vi "市电监测-自动重合闸.vi"() -> ()   [LabVIEW 2016, in "环境动力监测库.lvlib" / "自动重合闸库.lvlib"]
uses:
  <vilib>/Utility/miscctls.llb/LVPointTypeDef.ctl
panel:
  out "data":T1
  out "x+1":u32
  in  "解除告警":bool
  out "日用电量":dbl format="%#.1f"
  out "小时用电量":dbl format="%#.1f"
  in  "清零":bool
  out "累计用电量":dbl format="%#.1f"
  out "漏电报警累加值":u16 caption="漏电报警次数"
  out "当前报警状态":u16(ring) items=["无报警"=0, "过压报警"=1, "欠压报警"=2, "过流报警"=4, "漏电报警"=8]
  out "通讯状态":u16(ring) items=["正常", "异常"]
  out "过流报警累加值":u16 caption="过流报警次数"
  out "欠压报警累加值":u16 caption="欠压报警次数"
  out "过压报警累加值":u16 caption="过压报警次数"
  out "当前漏电电流":dbl
  out "当前电流":dbl
  out "当前电压":u16
  # "市电监测/自动重合闸"
  # "V"
  # "A"
  # "mA"
  # "KW·h"
  # "KW·h"
  # "KW·h"
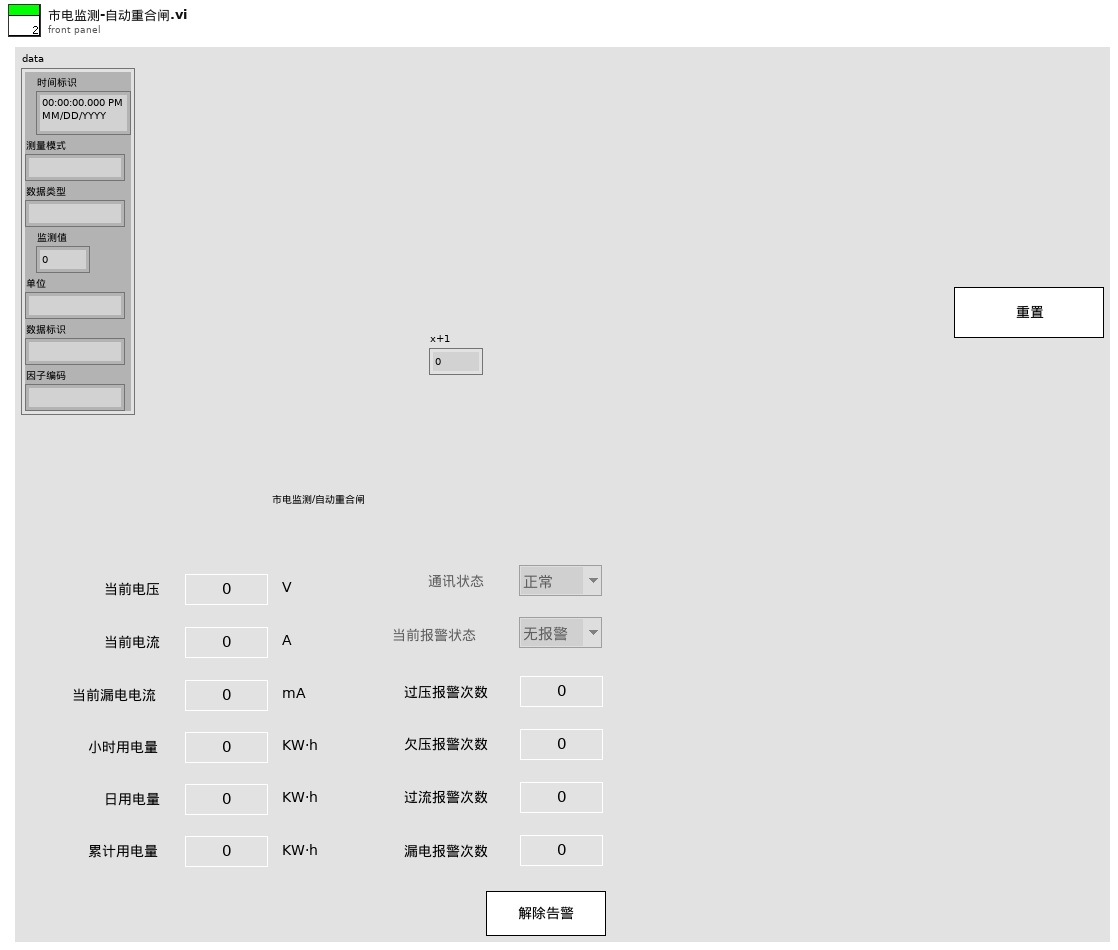
[diagram p1: front panel]
types:
  T1 = cluster{"时间标识":timestamp, "测量模式":string, "数据类型":string, "监测值":sgl, "单位":string, "数据标识":string, "因子编码":string}
  T2 = typedef "LVPointTypeDef.ctl" = cluster{"Horizontal":i16, "Vertical":i16}
  T3 = cluster{"监测项描述:输出":string, "端口":enum16{"AI0", "AI1", "AI2", "AI3", "AI4", "DI0", "DI1", "DI2", "DI3", "DI4", "DI5", "DI6", "DI7", "DO0", "DO1", "DO2", "DO3", "DO4", "DO5", "DO6", "DO7", "X0", "X1", "X2", "X3", "X4", "X5", "X6", "X7", "X8", "X9", "X10", "X11", "X12", "X13", "X14", "X15", "X16", "X17", "X18", "X19", "X20", "X21", "X22", "X23", "Y0", "Y1", "Y2", "Y3", "Y4", "Y5", "Y6", "Y7", "Y8", "Y9", "Y10", "Y11", "Y12", "Y13", "Y14", "Y15", "Y16", "Y17", "Y18", "Y19", "Y20", "Y21", "Y22", "Y23", "Y24", "Y25", "Y26", "Y27", "Y28", "Y29", "Y30", "Y31", "Y32", "Y33", "Y34", "Y35", "Y36", "Y37", "Y38", "Y39"}, "告警方式":enum32{"禁用告警", "闭合告警", "断开告警"}, "传感器型号":enum16{"PLC", "ZLAN", "ART"}, "声光告警启用":bool}
  T4 = enum16{"AI0", "AI1", "AI2", "AI3", "AI4", "DI0", "DI1", "DI2", "DI3", "DI4", "DI5", "DI6", "DI7", "DO0", "DO1", "DO2", "DO3", "DO4", "DO5", "DO6", "DO7", "X0", "X1", "X2", "X3", "X4", "X5", "X6", "X7", "X8", "X9", "X10", "X11", "X12", "X13", "X14", "X15", "X16", "X17", "X18", "X19", "X20", "X21", "X22", "X23", "Y0", "Y1", "Y2", "Y3", "Y4", "Y5", "Y6", "Y7", "Y8", "Y9", "Y10", "Y11", "Y12", "Y13", "Y14", "Y15", "Y16", "Y17", "Y18", "Y19", "Y20", "Y21", "Y22", "Y23", "Y24", "Y25", "Y26", "Y27", "Y28", "Y29", "Y30", "Y31", "Y32", "Y33", "Y34", "Y35", "Y36", "Y37", "Y38", "Y39"}
  T5 = cluster{"状态":cluster{"R0":i16, "R1":i16, "R2":i16, "R3":i16, "R4":i16, "R5":i16, "R6":i16, "R7":i16, "R8":i16, "R9":i16, "R10":i16, "R11":i16, "R12":i16, "R13":i16, "R14":i16, "R15":i16, "R16":i16, "R17":i16, "R18":i16, "R19":i16, "R20":i16, "R21":i16, "R22":i16, "R23":i16, "R24":i16, "R25":i16, "R26":i16, "R27":i16, "R28":i16, "R29":i16, "R30":i16, "R31":i16, "R32":i16, "R33":i16, "R34":i16, "R35":i16, "R36":i16, "R37":i16, "R38":i16, "R39":i16}, "输入状态":bool[], "输出状态":bool[], "参数设置":cluster{"R100":i16, "R101":i16, "R102":i16, "R103":i16, "R104":i16, "R105":i16, "R106":i16, "R107":i16, "R108":i16, "R109":i16, "R110":i16, "R111":i16, "R112":i16, "R113":i16, "R114":i16, "R115":i16, "R116":i16, "R117":i16, "R118":i16, "R119":i16, "R120":i16, "R121":i16, "R122":i16, "R123":i16}, "转换值":cluster{"AD0":sgl, "AD1":sgl, "AD2":sgl, "AD3":sgl, "AD4":sgl, "AD5":sgl}}
  T6 = cluster{"R0":i16, "R1":i16, "R2":i16, "R3":i16, "R4":i16, "R5":i16, "R6":i16, "R7":i16, "R8":i16, "R9":i16, "R10":i16, "R11":i16, "R12":i16, "R13":i16, "R14":i16, "R15":i16, "R16":i16, "R17":i16, "R18":i16, "R19":i16, "R20":i16, "R21":i16, "R22":i16, "R23":i16, "R24":i16, "R25":i16, "R26":i16, "R27":i16, "R28":i16, "R29":i16, "R30":i16, "R31":i16, "R32":i16, "R33":i16, "R34":i16, "R35":i16, "R36":i16, "R37":i16, "R38":i16, "R39":i16}
  T7 = typedef "采配水类型.ctl" = enum16{"V1", "V2", "V3", "V4", "室内V1", "室内V2", "固定站V1", "固定站V2", "浮船V1", "浮船V2", "养殖尾水", "广东华南所"}
  T8 = cluster{"状态":cluster{"R0":i16, "R1":i16, "R2":i16, "R3":i16, "R4":i16, "R5":i16, "R6":i16, "R7":i16, "R8":i16, "R9":i16, "R10":i16, "R11":i16, "R12":i16, "R13":i16, "R14":i16, "R15":i16, "R16":i16, "R17":i16, "R18":i16, "R19":i16, "R20":i16, "R21":i16, "R22":i16, "R23":i16, "R24":i16, "R25":i16, "R26":i16, "R27":i16, "R28":i16, "R29":i16, "R30":i16, "R31":i16, "R32":i16, "R33":i16, "R34":i16, "R35":i16, "R36":i16, "R37":i16, "R38":i16, "R39":i16, "R40":i16, "R41":i16, "R42":i16, "R43":i16, "R44":i16, "R45":i16, "R46":i16, "R47":i16, "R48":i16, "R49":i16, "R50":i16, "R51":i16, "R52":i16, "R53":i16, "R54":i16, "R55":i16, "R56":i16, "R57":i16, "R58":i16, "R59":i16, "R60":i16, "R61":i16, "R62":i16, "R63":i16, "R64":i16, "R65":i16, "R66":i16, "R67":i16, "R68":i16, "R69":i16}, "输入状态":bool[], "输出状态":bool[], "报警簇":bool[], "参数设置":cluster{"R100":i16, "R101":i16, "R102":i16, "R103":i16, "R104":i16, "R105":i16, "R106":i16, "R107":i16, "R108":i16, "R109":i16, "R110":i16, "R111":i16, "R112":i16, "R113":i16, "R114":i16, "R115":i16, "R116":i16, "R117":i16, "R118":i16, "R119":i16, "R120":i16, "R121":i16, "R122":i16, "R123":i16, "R124":i16}, "转换值":cluster{"AD0":sgl, "AD1":sgl, "AD2":sgl, "AD3":sgl, "AD4":sgl, "AD5":sgl}, "看门狗启用":bool, "氨氮模块名称":string, "总磷模块名称":string, "采配水模块类型":T7}
  T9 = cluster{"R0":i16, "R1":i16, "R2":i16, "R3":i16, "R4":i16, "R5":i16, "R6":i16, "R7":i16, "R8":i16, "R9":i16, "R10":i16, "R11":i16, "R12":i16, "R13":i16, "R14":i16, "R15":i16, "R16":i16, "R17":i16, "R18":i16, "R19":i16, "R20":i16, "R21":i16, "R22":i16, "R23":i16, "R24":i16, "R25":i16, "R26":i16, "R27":i16, "R28":i16, "R29":i16, "R30":i16, "R31":i16, "R32":i16, "R33":i16, "R34":i16, "R35":i16, "R36":i16, "R37":i16, "R38":i16, "R39":i16, "R40":i16, "R41":i16, "R42":i16, "R43":i16, "R44":i16, "R45":i16, "R46":i16, "R47":i16, "R48":i16, "R49":i16, "R50":i16, "R51":i16, "R52":i16, "R53":i16, "R54":i16, "R55":i16, "R56":i16, "R57":i16, "R58":i16, "R59":i16, "R60":i16, "R61":i16, "R62":i16, "R63":i16, "R64":i16, "R65":i16, "R66":i16, "R67":i16, "R68":i16, "R69":i16}
  T10 = cluster{"市电":cluster{"状态":bool, "电压:":u16, "电流：":dbl, "详情  ":bool}, "UPS":cluster{"状态":bool, "输入电压:":sgl, "输出电压:":sgl, "电池电量:":u8, "电量":u16, "详情  ":bool}, "蓄电池12V":cluster{"状态":bool, "电压:":sgl, "电流:":sgl, "电池电量:":u8, "电量":u16, "详情  ":bool, "充电":bool, "负载":bool}, "蓄电池24V":cluster{"状态":bool, "电压:":sgl, "电流:":sgl, "电池电量:":u8, "电量":u16, "详情  ":bool, "充电":bool, "负载":bool}}
  T11 = cluster{"漏水监测输出":cluster{"漏水监测告警":bool, "告警内容":string}, "门禁监测输出":cluster{"门禁监测告警":bool, "告警内容":string}, "门禁监测输出2":cluster{"门禁监测告警":bool, "告警内容":string}, "温湿度监测输出":cluster{"温湿度监测告警":bool, "告警内容":string}, "烟雾监测输出":cluster{"烟雾监测告警":bool, "告警内容":string}, "空调监测输出":cluster{"空调监测告警":bool, "告警内容":string}, "自动重合闸输出":cluster{"自动重合闸告警":bool, "告警内容":string}, "红外入侵输出":cluster{"红外入侵告警":bool, "告警内容":string}, "振动输出":cluster{"振动告警":bool, "告警内容":string}, "UPS输出":cluster{"UPS告警":bool, "告警内容":string}, "蓄电池输出":cluster{"蓄电池告警":bool, "告警内容":string}, "蓄电池输出2":cluster{"蓄电池告警":bool, "告警内容":string}, "GPS输出":cluster{"定位告警":bool, "告警内容":string}, "北斗输出":cluster{"定位告警":bool, "告警内容":string}, "气象输出":cluster{"气象告警":bool, "告警内容":string}, "废液输出":cluster{"废液告警":bool, "告警内容":string}, "废液输出2":cluster{"废液告警":bool, "告警内容":string}}
  T12 = typedef "LVDateTimeRec.ctl" = cluster{"秒数的小数部分":dbl, "秒":i32, "分":i32, "时":i32, "日":i32, "月":i32, "年":i32, "天数（周）":i32, "天数（年）":i32, "DST":i32}
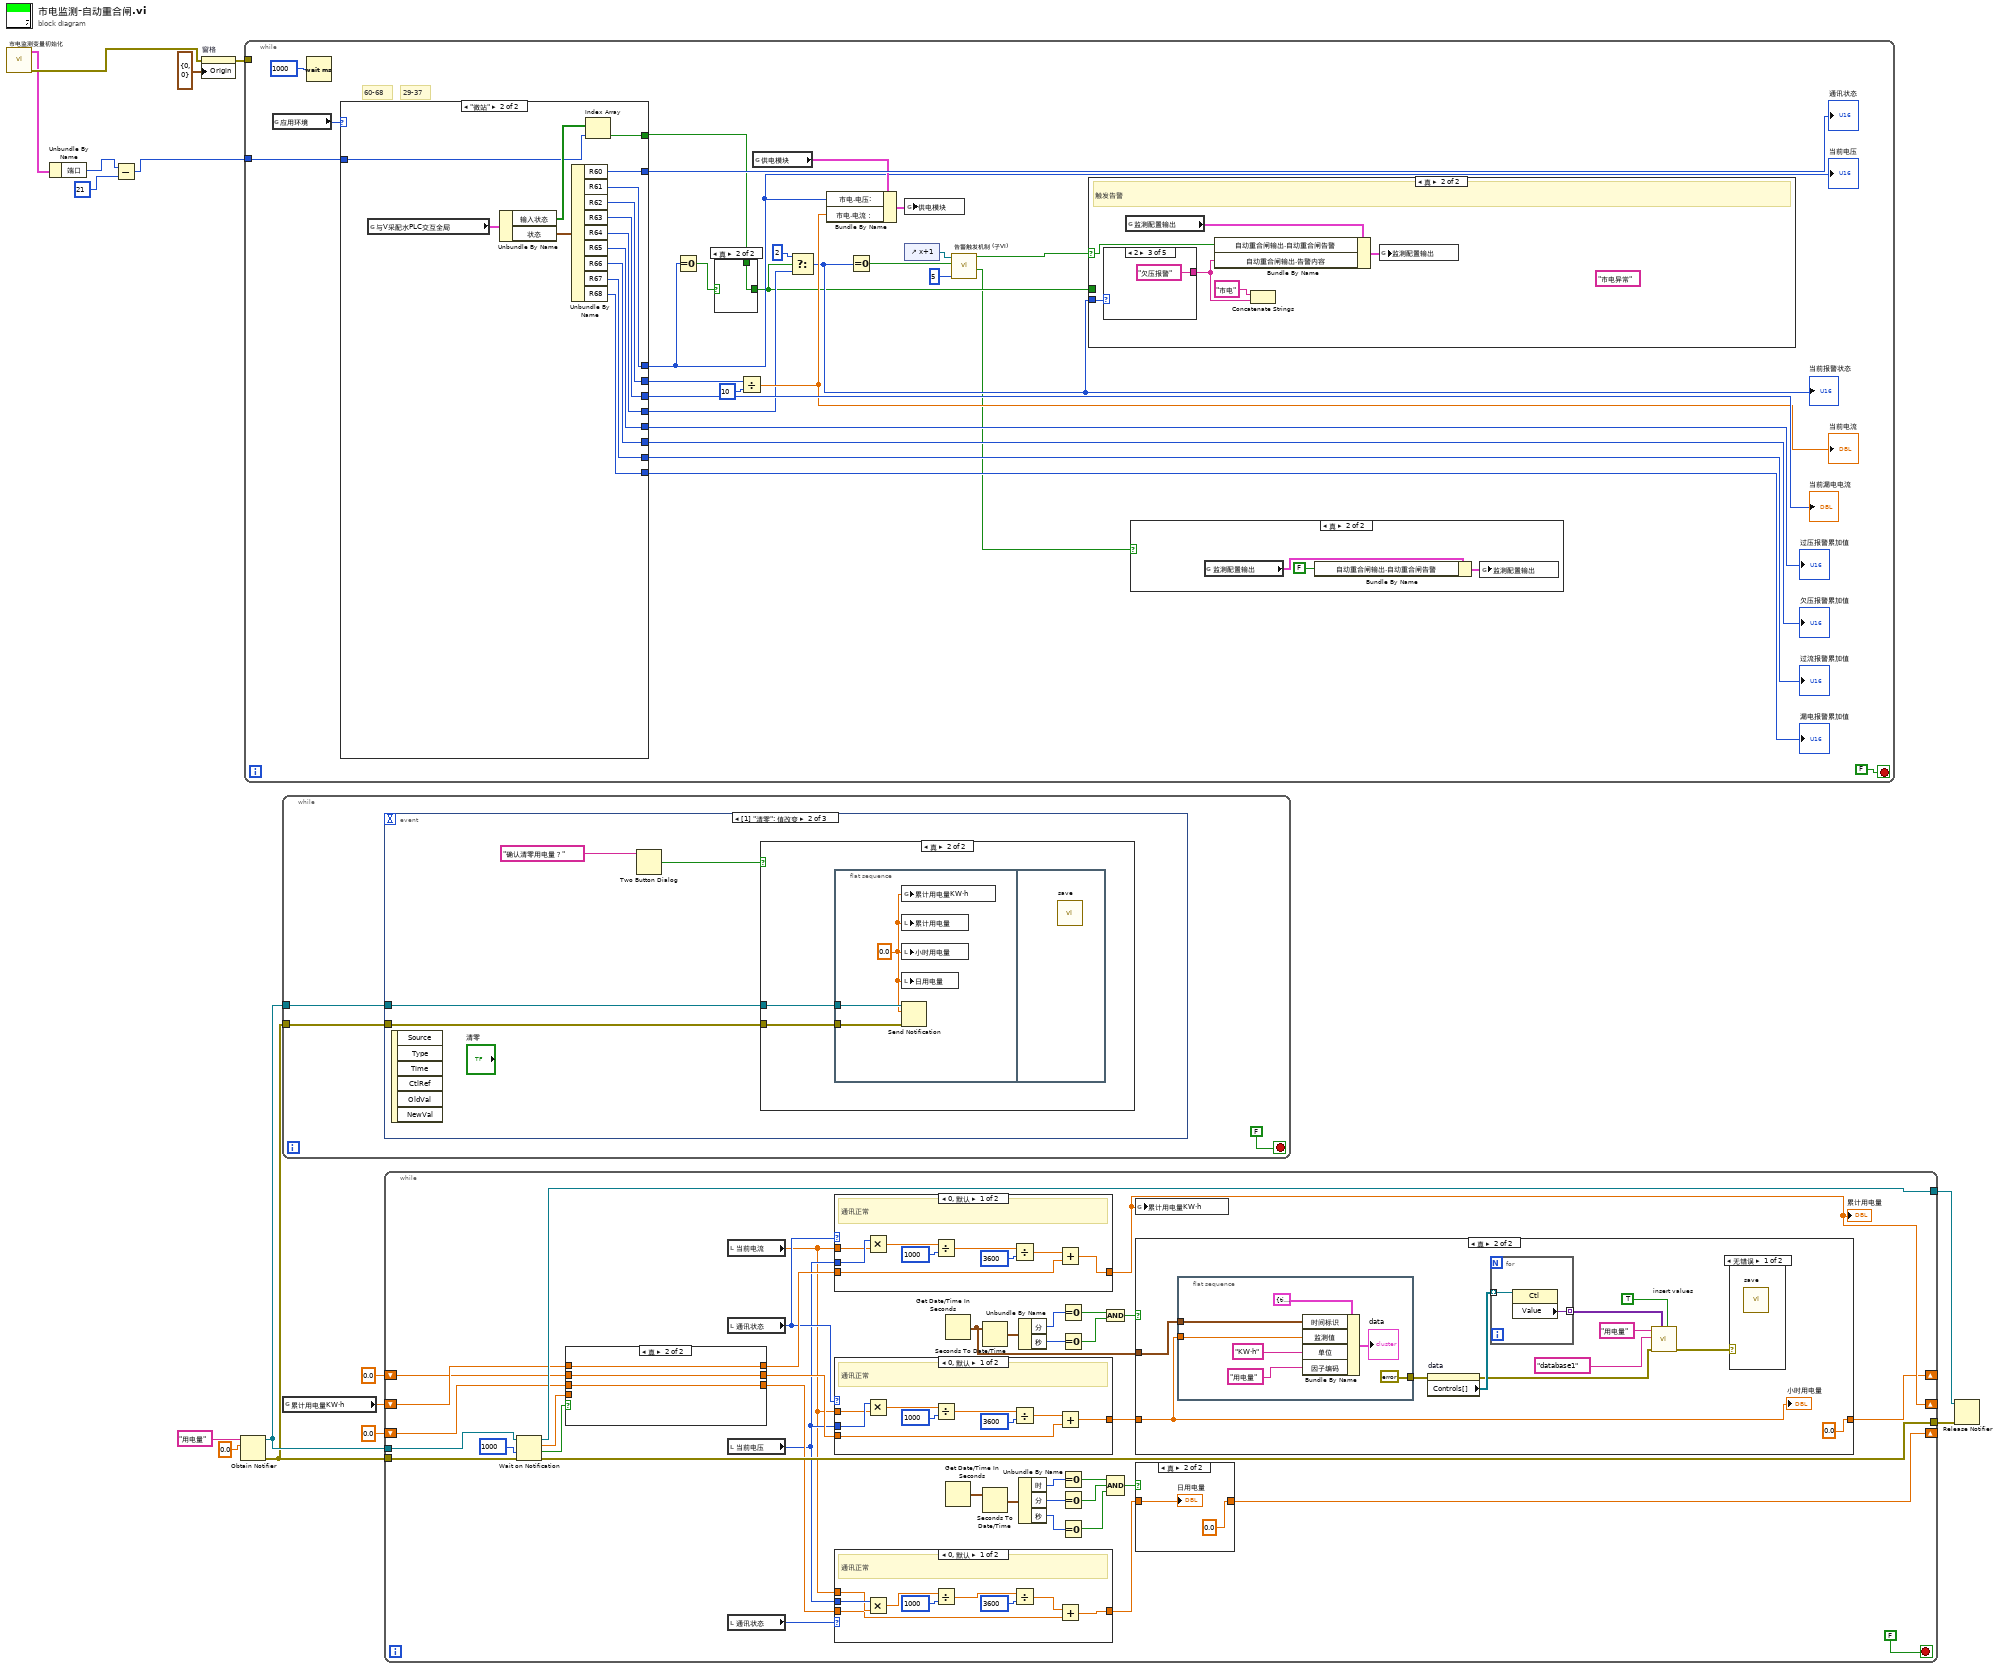
[diagram p0: block diagram]
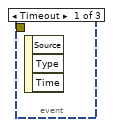
[diagram p9: hidden frame]
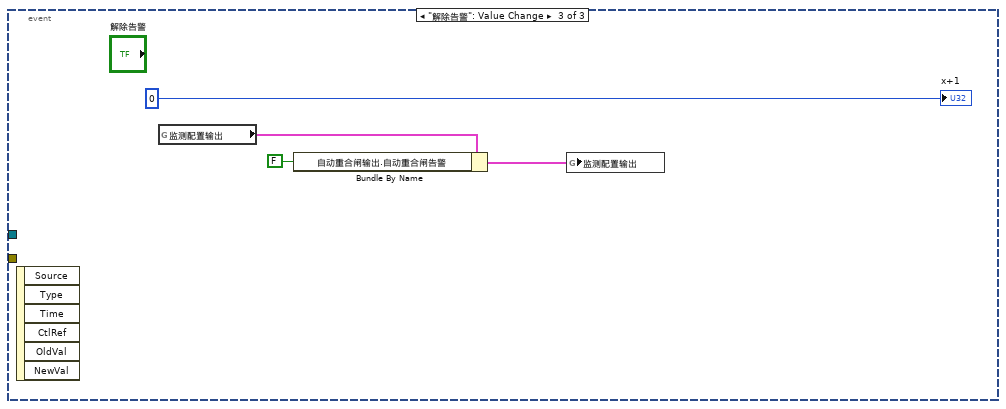
[diagram p11: hidden frame]
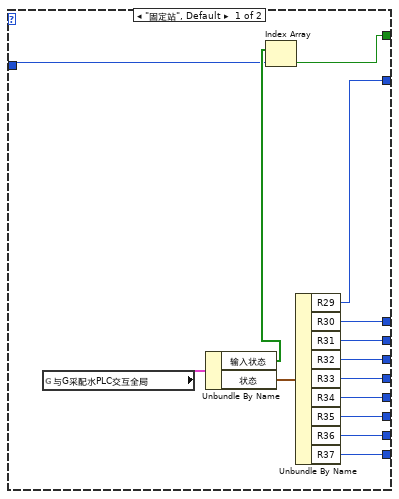
[diagram p14: hidden frame]
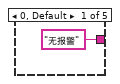
[diagram p16: hidden frame]
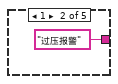
[diagram p17: hidden frame]
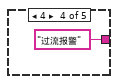
[diagram p18: hidden frame]
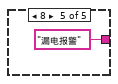
[diagram p19: hidden frame]
diagram:
  n1 = call "市电监测变量初始化.vi"() -> ("error out"=w5:errorcluster, "数据"=w4:T3)  [unwired: 10 in]
  n2 = Unbundle By Name(w4) -> ("端口"=w3:T4)
  n3 = Subtract(x=w3, y=21) -> (x-y=w1:i32)
  n4 = property on="窗格" class="Pane"(error in=w5, "Origin"=T2 {"Horizontal"=0, "Vertical"=0} ("原点")) -> (error out=w15:errorcluster)  [unwired: 1 in, 1 out]
  n5 = Obtain Notifier(name (unnamed)="用电量" ("名称（未命名）"), notification data type=0.0 ("y")) -> (notifier out=w12:refnum<notifier>, error out=w11:errorcluster)  [unwired: 2 in, 1 out]
  n6 = while {
    tunnel: w15 -> [_]
    tunnel: w1 -> [w21]
    stop <- FALSE stop-if-true
    # "60-68"
    # "29-37"
    n7 = global read "外部交互全局变量.vi" "应用环境"() -> (w40:enum16{"固定站", "微站", "浮标", "浮船"})
    n8 = Wait (ms)(milliseconds to wait=u32 1000 ("等待时间（毫秒）")) -> ()  [unwired: 1 out]
    n9 = case shown="\"微站\"" w40 {
      tunnel: [w60 w74] -> w39
      tunnel: [w59 w73] -> w27
      tunnel: [w58 w72] -> w38
      tunnel: [w57 w71] -> w37
      tunnel: [w56 w70] -> w25
      tunnel: [w55 w69] -> w36
      tunnel: [w54 w68] -> w35
      tunnel: [w53 w67] -> w34
      tunnel: [w52 w66] -> w33
      tunnel: [w49 w64] -> w19
      tunnel: w21 -> [w50 w63]
      frame "固定站", Default {
        n10 = global read "外部交互全局变量.vi" "与G采配水PLC交互全局"() -> (w62:T5)
        n11 = Unbundle By Name(w62) -> ("输入状态"=w51:bool[], "状态"=w61:T6)
        n12 = Index Array(array=w51, index=w50) -> (element=w49:bool)
        n13 = Unbundle By Name(w61) -> ("R29"=w60:i16, "R30"=w59:i16, "R31"=w58:i16, "R32"=w57:i16, "R33"=w56:i16, "R34"=w55:i16, "R35"=w54:i16, "R36"=w53:i16, "R37"=w52:i16)
      }
      frame "微站" {
        n14 = global read "外部交互全局变量.vi" "与V采配水PLC交互全局"() -> (w76:T8)
        n15 = Unbundle By Name(w76) -> ("输入状态"=w65:bool[], "状态"=w75:T9)
        n16 = Unbundle By Name(w75) -> ("R60"=w74:i16, "R61"=w73:i16, "R62"=w72:i16, "R63"=w71:i16, "R64"=w70:i16, "R65"=w69:i16, "R66"=w68:i16, "R67"=w67:i16, "R68"=w66:i16)
        n17 = Index Array(array=w65, index=w63) -> (element=w64:bool)
      }
    }
    "通讯状态" <- w39
    "当前电压" <- w27
    "当前漏电电流" <- w37
    "过压报警累加值" <- w36
    "欠压报警累加值" <- w35
    "过流报警累加值" <- w34
    "漏电报警累加值" <- w33
    n18 = Equal To 0?(x=w27) -> (x = 0?=w20:bool)
    n19 = case shown="真" w20 {
      selector: w20 -> [w47 _]
      tunnel: [w47 w48] -> w18
      tunnel: w19 -> [_ w48]
      frame False {
      }
      frame True {
      }
    }
    n20 = Divide(x=w38, y=i16 10) -> (x/y=w30:dbl)
    "当前电流" <- w30
    n21 = global read "内部交互全局变量.vi" "供电模块"() -> (w32:T10)
    n22 = Select(t=i16 2, s=w18, f=w25) -> (s? t:f=w24:i16)
    "当前报警状态" <- w24
    n23 = Bundle By Name(cluster=w32, "市电.电压:"=w27, "市电.电流："=w30) -> (w31:T10)
    n24 = Equal To 0?(x=w24) -> (x = 0?=w23:bool)
    n25 = global write "内部交互全局变量.vi" "供电模块"(w31) -> ()
    n26 = control-ref of="x+1"() -> (w29:refnum<vi>)
    n27 = call "告警触发机制 (子VI).vi"("信号持续时间"=u32 5, "状态输出真-正常"=w23, "Digital输入"=w29) -> ("消除告警"=w17:bool, "触发告警"=w22:bool)  [unwired: 6 in, 1 out]
    n28 = case shown="真" w22 {
      selector: w22 -> [_ w82]
      tunnel: w24 -> [_ w81]
      tunnel: w18 -> [_ _]
      frame False {
      }
      frame True {
        (unwired) "市电异常" ("设备")
        # "触发告警"
        n29 = case shown="2" w81 {
          tunnel: ["无报警" ("日志信息") "过压报警" ("日志信息") "欠压报警" ("日志信息") "过流报警" ("日志信息") "漏电报警" ("日志信息")] -> w79
          frame 0, Default {
          }
          frame 1 {
          }
          frame 2 {
          }
          frame 4 {
          }
          frame 8 {
          }
        }
        n30 = global read "内部交互全局变量.vi" "监测配置输出"() -> (w78:T11)
        n31 = Bundle By Name(cluster=w78, "自动重合闸输出.自动重合闸告警"=w82, "自动重合闸输出.告警内容"=w79) -> (w77:T11)
        n32 = Concatenate Strings("市电" ("报警内容"), w79) -> ()  [unwired: 1 out]
        n33 = global write "内部交互全局变量.vi" "监测配置输出"(w77) -> ()
      }
    }
    n34 = case shown="真" w17 {
      frame False {
      }
      frame True {
        n35 = global read "内部交互全局变量.vi" "监测配置输出"() -> (w45:T11)
        n36 = Bundle By Name(cluster=w45, "自动重合闸输出.自动重合闸告警"=FALSE) -> (w46:T11)
        n37 = global write "内部交互全局变量.vi" "监测配置输出"(w46) -> ()
      }
    }
  }
  n38 = while {
    tunnel: w12 -> [w90]
    tunnel: w11 -> [w89]
    stop <- FALSE stop-if-true
    n39 = event shown="[1] \"清零\": 值改变" {
      selector: _ -> [_ _ _]
      dyn-events: _ -> [_ _ _]
      timeout: _ -> [_ _ _]
      tunnel: w90 -> [_ w92 _]
      tunnel: w89 -> [_ w91 _]
      event Timeout {
        n40 = event-data() -> ()  [unwired: 1 in, 3 out]
      }
      event "清零": Value Change {
        n41 = event-data() -> ()  [unwired: 1 in, 6 out]
        n42 = Two Button Dialog(message="确认清零用电量？" ("消息")) -> (T button?=w93:bool)  [unwired: 2 in]
        n43 = case shown="真" w93 {
          tunnel: w92 -> [_ w96]
          tunnel: w91 -> [_ w95]
          frame False {
          }
          frame True {
            n44 = flat-sequence {
              tunnel: w96 -> [w99]
              tunnel: w95 -> [w98]
              frame #0 {
                w97 = 0.0 ("累计用电量KW/h")
                n45 = global write "断电保存全局变量.vi" "累计用电量KW·h"(w97) -> ()
                n46 = local write "累计用电量"(w97) -> ()
                n47 = local write "小时用电量"(w97) -> ()
                n48 = local write "日用电量"(w97) -> ()
                n49 = Send Notification(notification=w97, notifier=w99, error in (no error)=w98) -> ()  [unwired: 2 out]
              }
              frame #1 {
                n50 = call "save.vi"() -> ()  [unwired: 11 in, 1 out]
              }
            }
          }
        }
      }
      event "解除告警": Value Change {
        n51 = event-data() -> ()  [unwired: 1 in, 6 out]
        n52 = global read "内部交互全局变量.vi" "监测配置输出"() -> (w101:T11)
        n53 = Bundle By Name(cluster=w101, "自动重合闸输出.自动重合闸告警"=FALSE) -> (w100:T11)
        n54 = global write "内部交互全局变量.vi" "监测配置输出"(w100) -> ()
        "x+1" <- u32 0 ("x+1")
      }
    }
  }
  n55 = global read "断电保存全局变量.vi" "累计用电量KW·h"() -> (w8:dbl)
  n56 = while {
    tunnel: w12 -> [w141]
    tunnel: w11 -> [w140]
    tunnel: [w139] -> w10
    tunnel: [w138] -> w9
    shift-right: [w110] -> _
    shift-left: w8 -> [w137]
    shift-right: [w115] -> _
    shift-left: 0.0 -> [w112]
    shift-right: [w109] -> _
    shift-left: 0.0 -> [w113]
    stop <- FALSE stop-if-true
    n57 = Wait on Notification(notifier=w141, timeout in ms (-1)=1000 ("超时毫秒(-1)"), error in (no error)=w140) -> (notifier out=w139:refnum<notifier>, notification=w136:dbl, timed out?=w135:bool, error out=w138:errorcluster)  [unwired: 1 in]
    n58 = case shown="真" w135 {
      tunnel: [w197 w200] -> w134
      tunnel: w137 -> [_ w200]
      tunnel: [w197 w199] -> w107
      tunnel: w136 -> [w197 _]
      tunnel: w113 -> [_ w199]
      tunnel: w112 -> [_ w198]
      tunnel: [w197 w198] -> w111
      frame False {
      }
      frame True {
      }
    }
    n59 = local read "当前电流"() -> (w104:dbl)
    n60 = local read "通讯状态"() -> (w106:u16)
    n61 = local read "当前电压"() -> (w105:u16)
    n62 = local read "通讯状态"() -> (w118:u16)
    n63 = case shown="0, 默认" w106 {
      tunnel: w105 -> [w193 _]
      tunnel: w104 -> [w192 _]
      tunnel: w134 -> [w191 w196]
      tunnel: [w190 w196] -> w110
      frame 0, Default {
        # "通讯正常"
        n64 = Multiply(x=w193, y=w192) -> (x*y=w194:dbl)
        n65 = Divide(x=w194, y=1000) -> (x/y=w188:dbl)
        n66 = Divide(x=w188, y=3600) -> (x/y=w187:dbl)
        n67 = Add(x=w187, y=w191) -> (x+y=w190:dbl)
      }
      frame 1 {
        # "通信异常"
      }
    }
    "累计用电量" <- w110
    n68 = case shown="0, 默认" w106 {
      tunnel: w105 -> [w149 _]
      tunnel: w104 -> [w148 _]
      tunnel: w107 -> [w147 w152]
      tunnel: [w146 w152] -> w108
      frame 0, Default {
        # "通讯正常"
        n69 = Multiply(x=w149, y=w148) -> (x*y=w150:dbl)
        n70 = Divide(x=w150, y=1000) -> (x/y=w144:dbl)
        n71 = Divide(x=w144, y=3600) -> (x/y=w143:dbl)
        n72 = Add(x=w143, y=w147) -> (x+y=w146:dbl)
      }
      frame 1 {
        # "通信异常"
      }
    }
    n73 = case shown="0, 默认" w118 {
      tunnel: w105 -> [w162 _]
      tunnel: w104 -> [w161 _]
      tunnel: w111 -> [w160 w165]
      tunnel: [w159 w165] -> w116
      frame 0, Default {
        # "通讯正常"
        n74 = Multiply(x=w162, y=w161) -> (x*y=w163:dbl)
        n75 = Divide(x=w163, y=1000) -> (x/y=w157:dbl)
        n76 = Divide(x=w157, y=3600) -> (x/y=w156:dbl)
        n77 = Add(x=w156, y=w160) -> (x+y=w159:dbl)
      }
      frame 1 {
        # "通信异常"
      }
    }
    n78 = Get Date/Time In Seconds() -> (seconds since 1Jan1904=w127:timestamp)
    n79 = Get Date/Time In Seconds() -> (seconds since 1Jan1904=w126:timestamp)
    n80 = Seconds To Date/Time(time stamp (now)=w127) -> (date time rec=w129:T12)  [unwired: 1 in]
    n81 = Seconds To Date/Time(time stamp (now)=w126) -> (date time rec=w125:T12)  [unwired: 1 in]
    n82 = Unbundle By Name(w129) -> ("分"=w130:i32, "秒"=w131:i32)
    n83 = Unbundle By Name(w125) -> ("时"=w120:i32, "分"=w124:i32, "秒"=w123:i32)
    n84 = Equal To 0?(x=w130) -> (x = 0?=w132:bool)
    n85 = Equal To 0?(x=w131) -> (x = 0?=w133:bool)
    n86 = Equal To 0?(x=w120) -> (x = 0?=w119:bool)
    n87 = Equal To 0?(x=w124) -> (x = 0?=w122:bool)
    n88 = Equal To 0?(x=w123) -> (x = 0?=w121:bool)
    n89 = And(x=w132, y=w133) -> (x .and. y?=w128:bool)
    n90 = Compound Arithmetic op=AND ("复合运算")(w119, w122, w121) -> (w117:bool)
    n91 = global write "断电保存全局变量.vi" "累计用电量KW·h"(w110) -> ()
    n92 = case shown="真" w128 {
      tunnel: [w166 0.0 ("y")] -> w109
      tunnel: w108 -> [w166 w176]
      tunnel: w127 -> [_ w177]
      frame False {
      }
      frame True {
        n93 = flat-sequence {
          tunnel: w177 -> [w181]
          tunnel: w176 -> [w180]
          tunnel: [errorcluster {"status"=FALSE, "code"=0, "source"=""} ("错误输入（无错误）")] -> w168
          frame #0 {
            n94 = Bundle By Name(cluster=T1 {"时间标识"=timestamp(0 s since 1904-01-01), "测量模式"="水样测试", "数据类型"="N", "监测值"=0.0, "单位"="mg/L", "数据标识"="N", "因子编码"=""} ("data"), "时间标识"=w181, "监测值"=w180, "单位"="KW·h", "因子编码"="用电量") -> (→"data":T1)
          }
        }
        n95 = property on="data" class="Clust (严格)"(error in=w168) -> (error out=w167:errorcluster, "Controls[]"=w172:refnum<vi>[])  [unwired: 1 in, 1 out]
        n96 = for {
          tunnel: w172 -> [w186] mode=indexing
          tunnel: [w185] -> w171 mode=indexing
          n97 = property class="Ctl"(reference=w186) -> ("Value"=w185:variant)  [unwired: 1 in, 2 out]
        }
        n98 = call "insert values.vi"("是否创建唯一键"=TRUE, "data"=w171, "错误输入（无错误）"=w167, "database"="database1", "Tabe Name"="用电量" ("table")) -> ("错误输出"=w169:errorcluster)  [unwired: 6 in]
        n99 = case shown="无错误" w169 {
          frame No Error {
            n100 = call "save.vi"() -> ()  [unwired: 11 in, 1 out]
          }
          frame Error {
          }
        }
        "小时用电量" <- w176
      }
    }
    n101 = case shown="真" w117 {
      tunnel: w116 -> [w153 w155]
      tunnel: [w153 0.0] -> w115
      frame False {
      }
      frame True {
        "日用电量" <- w155
      }
    }
  }
  n102 = Release Notifier(notifier=w10, error in (no error)=w9) -> ()  [unwired: 1 in, 3 out]
